vi "Initialize View.vi"(8 "error in (no error)":errorcluster, 9 "Refresh rate":i32, 10 "URL":string, 11 "Message Queues in":T1) -> (0 "error out":errorcluster, 3 "dup Message Queues":T1)   [LabVIEW 2023, in "Weather Monitor Views.lvlib"]
doc: "Initializes the message loops in preparation of starting a new view."
uses:
  Weather Monitor Views.lvlib
  support/Message Queue/All Message Queues.ctl
  support/Message Queue/Message Cluster.ctl
  support/Message Queue/Weather Message Queue.lvlib
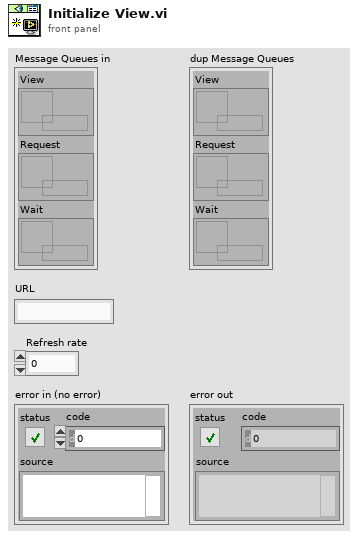
[diagram p1: front panel]
types:
  T1 = typedef "Weather Message Queue.lvlib/All Message Queues.ctl" = cluster{"View":refnum<queue>, "Request":refnum<queue>, "Wait":refnum<queue>}
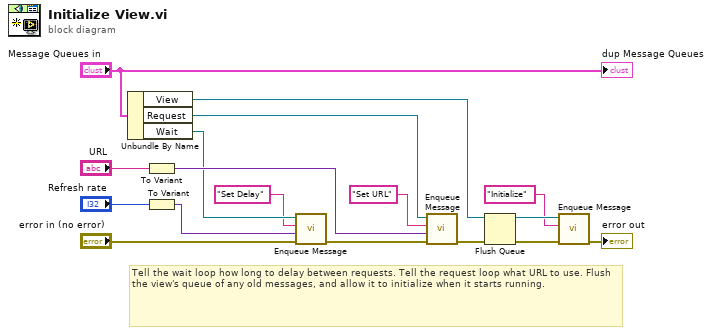
[diagram p0: block diagram]
diagram:
  # "Tell the wait loop how long to delay between requests. Tell the request loop what URL to use. Flush the view's queue of any old messages, and allow it to initialize when it starts running."
  n1 = Unbundle By Name("Message Queues in") -> ("View"=w2:refnum<queue>, "Request"=w12:refnum<queue>, "Wait"=w9:refnum<queue>)
  n2 = To Variant(anything="URL") -> (Variant=w13:variant)
  n3 = To Variant(anything="Refresh rate") -> (Variant=w11:variant)
  n4 = call "Enqueue Message.vi"("error in (no error)"="error in (no error)", "Message Data"=w11, "Message"="Set Delay", "Message Queue"=w9) -> ("error out"=w4:errorcluster)  [unwired: 6 in, 1 out]
  n5 = call "Enqueue Message.vi"("error in (no error)"=w4, "Message Data"=w13, "Message"="Set URL", "Message Queue"=w12) -> ("error out"=w3:errorcluster)  [unwired: 6 in, 1 out]
  n6 = Flush Queue(queue=w2, error in (no error)=w3) -> (queue out=w16:refnum<queue>, error out=w17:errorcluster)  [unwired: 1 out]
  n7 = call "Enqueue Message.vi"("error in (no error)"=w17, "Message"="Initialize", "Message Queue"=w16) -> ("error out"=→"error out":errorcluster)  [unwired: 7 in, 1 out]
  "dup Message Queues" <- "Message Queues in"
